vi "Calculate Normal Array.vi"(8 "error in (no error)":errorcluster, 9 "Coordinates System":enum16{"Cartesian", "Cylindrical", "Spherical"}(ring), 10 "3D Quiver Datatype.lvclass in":refnum<class "3D Quiver Datatype.lvclass">, 11 "Plot Representation In":T1) -> (0 "error out":errorcluster, 1 "Dup Coordinates System":enum16{"Cartesian", "Cylindrical", "Spherical"}(ring), 2 "3D Quiver Datatype.lvclass out":refnum<class "3D Quiver Datatype.lvclass">, 3 "Plot Representation Out":T1)   [LabVIEW 2017, in "3D Quiver Datatype.lvclass"]
uses:
  <vilib>/Math Plots/3D Math Plots/3D Quiver/3D Quiver Datatype/3D Quiver Datatype.lvclass
  <vilib>/Math Plots/3D Math Plots/3D Plot/3D Plot/Typedef/Plot Representation.ctl
  <vilib>/Math Plots/3D Math Plots/3D Plot/3D Plot/Typedef/Range Clusters.ctl
  <vilib>/Math Plots/3D Math Plots/3D Plot/3D Plot/Typedef/Mesh Data.ctl
  <vilib>/Math Plots/3D Math Plots/3D Quiver/3D Quiver Datatype/3D Quiver Datatype.lvclass/3D Quiver Datatype.ctl
  <vilib>/Math Plots/3D Math Plots/3D Plot/3D Plot Datatype/3D Plot Datatype.lvclass
  <vilib>/Math Plots/3D Math Plots/3D Plot/3D Plot/3D Plot.lvclass
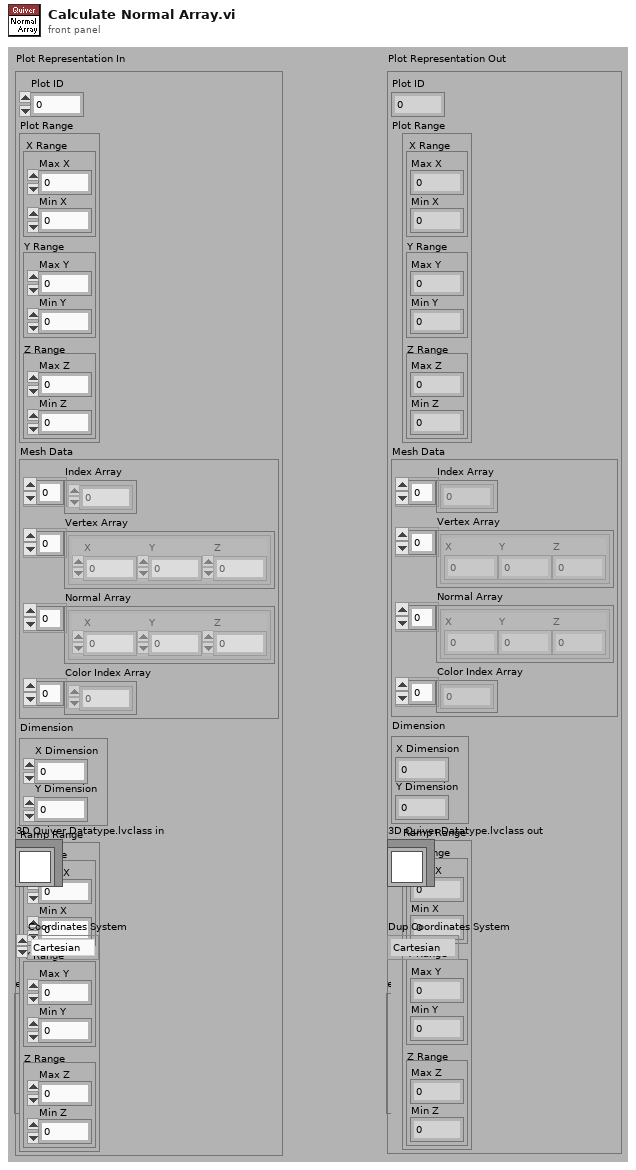
[diagram p1: front panel]
types:
  T1 = typedef "3D Plot.lvclass/Plot Representation.ctl" = cluster{"Plot ID":i32, "Plot Range":T2, "Mesh Data":T3, "Dimension":cluster{"X Dimension":i32, "Y Dimension":i32}, "Ramp Range":T2}
  T2 = typedef "3D Plot.lvclass/Range Clusters.ctl" = cluster{"X Range":cluster{"Max X":sgl, "Min X":sgl}, "Y Range":cluster{"Max Y":sgl, "Min Y":sgl}, "Z Range":cluster{"Max Z":sgl, "Min Z":sgl}}
  T3 = typedef "3D Plot.lvclass/Mesh Data.ctl" = cluster{"Index Array":u32[], "Vertex Array":cluster{"X":sgl, "Y":sgl, "Z":sgl}[], "Normal Array":cluster{"X":sgl, "Y":sgl, "Z":sgl}[], "Color Index Array":i32[]}
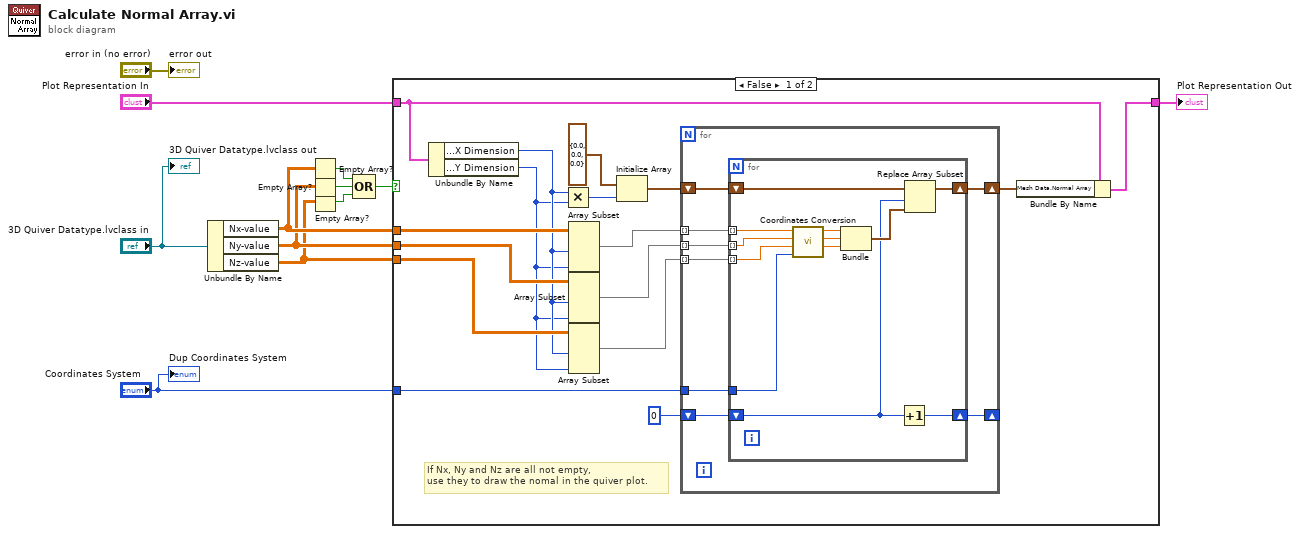
[diagram p0: block diagram]
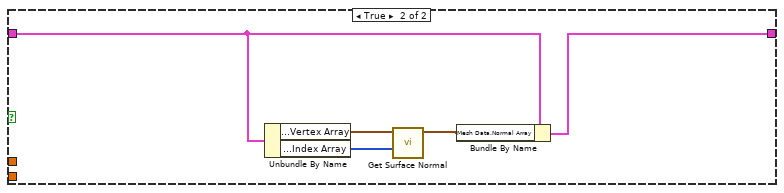
[diagram p2: hidden frame]
diagram:
  n1 = Unbundle By Name("3D Quiver Datatype.lvclass in") -> ("Nx-value"=w3:sgl[][], "Ny-value"=w2:sgl[][], "Nz-value"=w1:sgl[][])
  n2 = Empty Array?(array=w3) -> (empty?=w6:bool)
  n3 = Empty Array?(array=w2) -> (empty?=w7:bool)
  n4 = Empty Array?(array=w1) -> (empty?=w5:bool)
  n5 = Compound Arithmetic op=OR(w6, w7, w5) -> (w4:bool)
  n6 = case shown="False" w4 {
    tunnel: "Plot Representation In" -> [w18 w53]
    tunnel: [w27 w52] -> w11
    tunnel: w3 -> [w21 _]
    tunnel: w2 -> [w20 _]
    tunnel: w1 -> [w19 _]
    tunnel: "Coordinates System" -> [w26 _]
    frame False {
      # "If Nx, Ny and Nz are all not empty, \nuse they to draw the nomal in the quiver plot."
      n7 = Unbundle By Name(w18) -> ("Dimension.X Dimension"=w17:i32, "Dimension.Y Dimension"=w16:i32)
      n8 = Multiply(x=w17, y=w16) -> (x*y=w22:i32)
      n9 = Array Subset(array=w21, length (row)=w17, length (col)=w16) -> (w13:sgl[][])  [unwired: 2 in]
      n10 = Array Subset(array=w20, length (row)=w17, length (col)=w16) -> (w15:sgl[][])  [unwired: 2 in]
      n11 = Array Subset(array=w19, length (row)=w17, length (col)=w16) -> (w14:sgl[][])  [unwired: 2 in]
      n12 = Initialize Array(cluster{"X":sgl, "Y":sgl, "Z":sgl} {"X"=0.0, "Y"=0.0, "Z"=0.0} ("3D Point"), w22) -> (w24:cluster{"X":sgl, "Y":sgl, "Z":sgl}[])
      n13 = for {
        shift-right: [w35] -> w28
        shift-left: w24 -> [w36]
        tunnel: w14 -> [w34] mode=indexing
        tunnel: w13 -> [w32] mode=indexing
        tunnel: w15 -> [w33] mode=indexing
        tunnel: w26 -> [w31]
        shift-right: [w30] -> _
        shift-left: 0 -> [w29]
        n14 = for {
          tunnel: w34 -> [w46] mode=indexing
          shift-right: [w40] -> w35
          shift-left: w36 -> [w41]
          tunnel: w33 -> [w47] mode=indexing
          tunnel: w32 -> [w48] mode=indexing
          tunnel: w31 -> [w42]
          shift-right: [w38] -> w30
          shift-left: w29 -> [w37]
          n15 = call <vilib>:"Coordinates Conversion.vi"("Coordinates System"=w42, "Z in"=w46, "Y in"=w47, "X in"=w48) -> ("Z out"=w43:sgl, "Y out"=w44:sgl, "X out"=w45:sgl)  [unwired: 5 out]
          n16 = Bundle("X out"=w45, "Y out"=w44, "Z out"=w43) -> (w39:cluster{"X out":sgl, "Y out":sgl, "Z out":sgl})  [unwired: 1 out]
          n17 = Increment(x=w37) -> (x+1=w38:i32)
          n18 = Replace Array Subset(array=w41, new element=w39, index=w37) -> (w40:cluster{"X":sgl, "Y":sgl, "Z":sgl}[])
        }
      }
      n19 = Bundle By Name(cluster=w18, "Mesh Data.Normal Array"=w28) -> (w27:T1)
    }
    frame True {
      n20 = Unbundle By Name(w53) -> ("Mesh Data.Vertex Array"=w51:cluster{"X":sgl, "Y":sgl, "Z":sgl}[], "Mesh Data.Index Array"=w49:u32[])
      n21 = call <vilib>:"Get Surface Normal.vi"("Triangle Index Array"=w49, "Vertex Array"=w51) -> ("Normal Array"=w50:cluster{"X":sgl, "Y":sgl, "Z":sgl}[])  [unwired: 9 out]
      n22 = Bundle By Name(cluster=w53, "Mesh Data.Normal Array"=w50) -> (w52:T1)
    }
  }
  "Plot Representation Out" <- w11
  "error out" <- "error in (no error)"
  "3D Quiver Datatype.lvclass out" <- "3D Quiver Datatype.lvclass in"
  "Dup Coordinates System" <- "Coordinates System"
